vi "write ikon class.vi"(8 "error in (no error)":errorcluster, 10 "iKon-L.lvclass":refnum<class "iKon-L.lvclass">, 11 "SPARC4_Channel in":refnum<class "ECHARPE_Channel.lvclass">) -> (0 "error out":errorcluster, 3 "SPARC4_Channel out":refnum<class "ECHARPE_Channel.lvclass">)   [LabVIEW 2018, in "ECHARPE_Channel.lvclass"]
uses:
  ECHARPE_Channel.lvclass
  C:/Users/Denis/Desktop/S4ACS/S4ACS/Channel/Channel.lvclass
  iKon-L/iKon-L.lvclass
  C:/Users/Denis/Desktop/S4ACS/S4ACS/Sim_CCD/Sim_CCD.lvclass
  Channel/Channel.lvclass/Channel.ctl
  Channel/Channel.lvclass
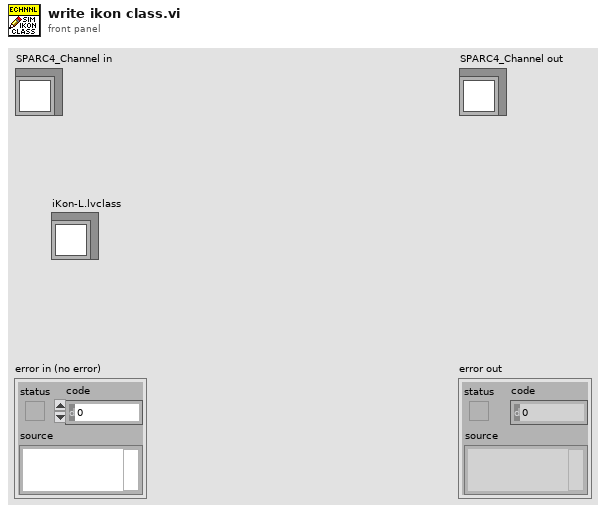
[diagram p1: front panel]
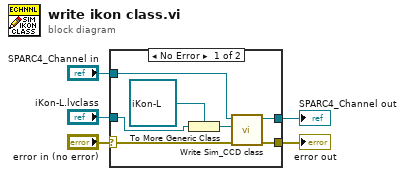
[diagram p0: block diagram]
diagram:
  n1 = case shown="No Error" "error in (no error)" {
    selector: "error in (no error)" -> [w10 w14]
    tunnel: [w9 w14] -> w4
    tunnel: [w11 w13] -> w2
    tunnel: "SPARC4_Channel in" -> [w12 w13]
    tunnel: "iKon-L.lvclass" -> [w8 _]
    frame No Error {
      n2 = To More Generic Class(target class=refnum<class "iKon-L.lvclass"> refnum ("iKon-L.lvclass"), reference=w8) -> (generic class reference=w7:refnum<class "iKon-L.lvclass">)
      n3 = call "Write Sim_CCD class.vi"("error in (no error)"=w10, "Sim_CCD.lvclass"=w7, "Channel in"=w12) -> ("error out"=w9:errorcluster, "Channel out"=w11:refnum<class "ECHARPE_Channel.lvclass">)  [unwired: 7 in]
    }
    frame Error {
    }
  }
  "error out" <- w4
  "SPARC4_Channel out" <- w2
